vi "LAC pharse Msg (SubVI).vi"(2 "result":string) -> (0 "array out":string[](array[string]), 1 "ERR?":bool)   [LabVIEW 2014]
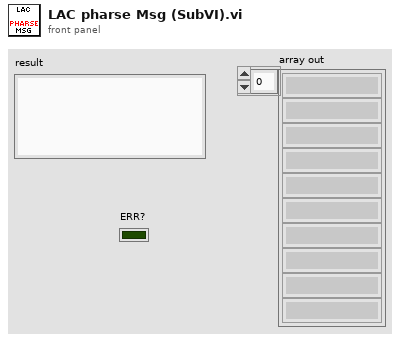
[diagram p1: front panel]
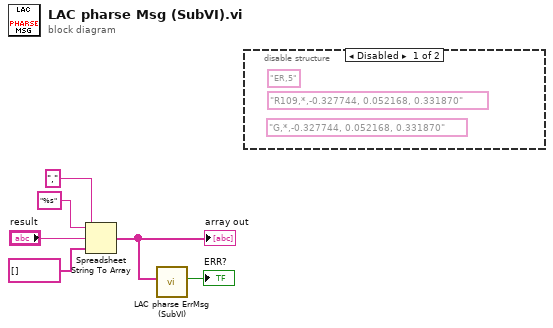
[diagram p0: block diagram]
diagram:
  n1 = Spreadsheet String To Array(delimiter (Tab)=",", format string="%s", spreadsheet string="result", array type (2D Dbl)=string[] []) -> (array=w2:string[])
  "array out" <- w2
  n2 = call "LAC pharse ErrMsg (SubVI).vi"("Response"=w2) -> ("ERR?"=→"ERR?":bool)  [unwired: 8 in, 2 out]
  n3 = disable-structure shown="Disabled" {
    frame Disabled {
      (unwired) "G,*,-0.327744, 0.052168, 0.331870"
      (unwired) "ER,5"
      (unwired) "R109,*,-0.327744, 0.052168, 0.331870"
    }
    frame Enabled {
    }
  }
